vi "textStyle.vi"() -> ()   [LabVIEW 2012]
panel:
  out "String out":string
  in  "String in":string
  in  "textSpec":T1
  in  "\"At\" location":T2
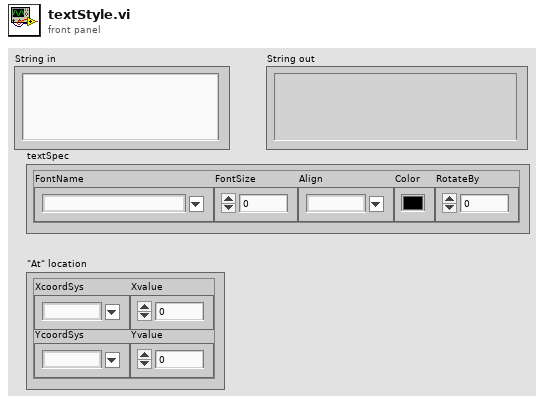
[diagram p1: front panel]
types:
  T1 = cluster{"FontName":string, "FontSize":u8, "Align":string, "Color":u32, "RotateBy":dbl}
  T2 = cluster{"XcoordSys":string, "YcoordSys":string, "Xvalue":dbl, "Yvalue":dbl}
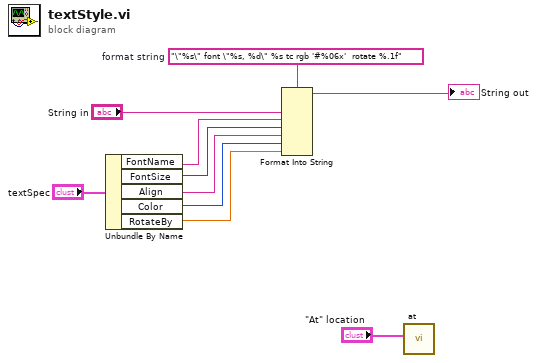
[diagram p0: block diagram]
diagram:
  w7 = "\"%s\" font \"%s, %d\" %s tc rgb '#%06x'  rotate %.1f"  # format string
  n1 = Unbundle By Name("textSpec") -> ("FontName"=w5:string, "FontSize"=w4:u8, "Align"=w3:string, "Color"=w2:u32, "RotateBy"=w1:dbl)
  n2 = Format Into String(format string=w7, "String in", w5, w4, w3, w2, w1) -> (resulting string=→"String out":string)  [unwired: 2 in, 1 out]
  n3 = call "at.vi"("\"At\" location"="\"At\" location") -> ()  [unwired: 10 in, 1 out]
